vi "Compute Time.vi"(8 "error in (no error)":errorcluster, 11 "Test Suite in":refnum<class "Test Suite.lvclass">) -> (0 "error out":errorcluster, 2 "Time":dbl, 3 "Test Suite out":refnum<class "Test Suite.lvclass">)   [LabVIEW 2013, in "JUnit XML.lvlib" / "Test Suite.lvclass"]
uses:
  Test Suite.lvclass
  Test Suite.lvclass/Test Suite.ctl
  Test Case/Test Case.lvclass/Test Case.ctl
  Test Case/Read Time.vi
  Test Case/Test Case.lvclass
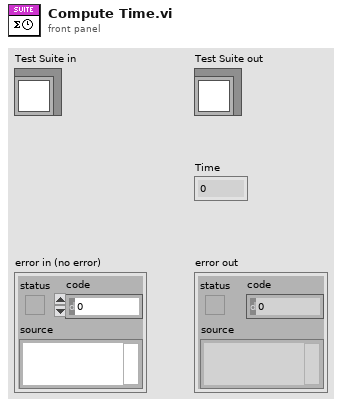
[diagram p1: front panel]
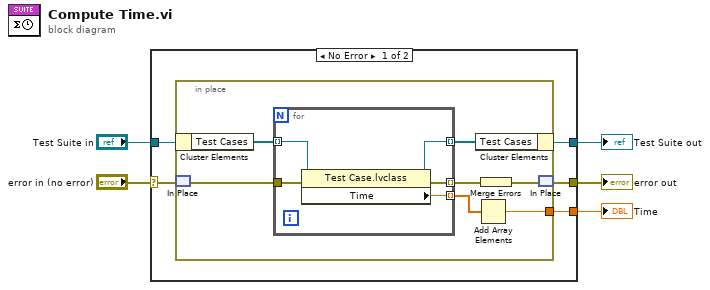
[diagram p0: block diagram]
diagram:
  n1 = case shown="No Error" "error in (no error)" {
    selector: "error in (no error)" -> [w7 w24]
    tunnel: [w6 w24] -> w4
    tunnel: [w9 w23] -> w2
    tunnel: "Test Suite in" -> [w10 w23]
    tunnel: [w8 _] -> w1
    frame No Error {
      n2 = in-place {
        in-place-border: [w14] -> w8
        n3 = in-place-cluster #1(w10) -> ("Test Cases"=w17:refnum<class "Test Case.lvclass">[])
        n4 = in-place-match #2(w7) -> (w13:errorcluster)
        n5 = for {
          tunnel: w17 -> [w22] mode=indexing
          tunnel: [w21] -> w16 mode=indexing
          tunnel: [w20] -> w15 mode=indexing
          tunnel: w13 -> [w19]
          tunnel: [w18] -> w12 mode=indexing
          n6 = property class="Test Case.lvclass"(reference=w22, error in=w19) -> (reference out=w21:refnum<class "Test Case.lvclass">, error out=w18:errorcluster, "Time"=w20:dbl)
        }
        n7 = in-place-cluster #1("Test Cases"=w16) -> (w9:refnum<class "Test Suite.lvclass">)
        n8 = Add Array Elements(numeric array=w15) -> (sum=w14:dbl)
        n9 = Merge Errors(w12) -> (w11:errorcluster)
        n10 = in-place-match #2(w11) -> (w6:errorcluster)
      }
    }
    frame Error {
    }
  }
  "error out" <- w4
  "Test Suite out" <- w2
  "Time" <- w1
